vi "byte2str.vi"(4 "byte":u8) -> (1 "String":string)   [LabVIEW 2015]
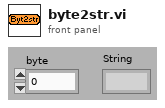
[diagram p1: front panel]
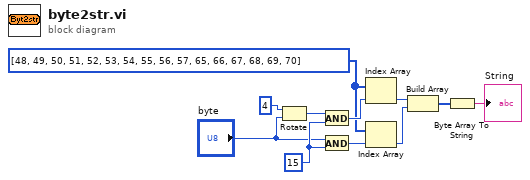
[diagram p0: block diagram]
diagram:
  w6 = u8[] [48, 49, 50, 51, 52, 53, 54, 55, 56, 57, 65, 66, 67, 68, 69, 70] ("byte Array")
  w10 = u8 15 ("y")
  n1 = Rotate(1:"byte", 2:i8 4 ("y")) -> (0:w9:u8)
  n2 = And(x=w9, y=w10) -> (x .and. y?=w8:u8)
  n3 = And(x="byte", y=w10) -> (x .and. y?=w7:u8)
  n4 = Index Array(array=w6, index=w8) -> (element=w4:u8)
  n5 = Index Array(array=w6, index=w7) -> (element=w3:u8)
  n6 = Build Array(w4, w3) -> (w2:u8[])
  n7 = Byte Array To String(unsigned byte array=w2) -> (string=→"String":string)
